vi "error result.vi"() -> (3 "result":refnum<class "result.lvclass">)   [LabVIEW 2013, in "result.lvclass"]
uses:
  result.lvclass
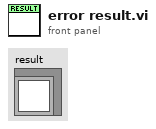
[diagram p1: front panel]
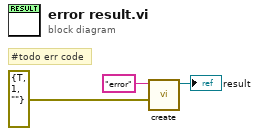
[diagram p0: block diagram]
diagram:
  # "#todo err code"
  n1 = call "create.vi"("error"=errorcluster {"status"=TRUE, "code"=1, "source"=""}, "data ID"="error") -> ("result out"=→"result":refnum<class "result.lvclass">)  [unwired: 9 in]
